vi "UDPrecieverShortLoop.vi"() -> ()   [LabVIEW 2012]
panel:
  out "Array":bool[][](array[boolean])
  out "size(s)":i32
  out "number":u32
  out "data pre process":u32
  out "packet in \nconstruction":u32
  out "data process":u32
  out "packet constructed":u32
  out "packet\nprocess":u32
  out "UDP reciever\nloop":u32
  out "start time":u32
  out "channel 11":u32[](graph)
  out "in 11":bool
  out "channel 10":u32[](graph)
  out "in 10":bool
  out "channel 9":u32[](graph)
  out "in 9":bool
  out "channel 8":u32[](graph)
  out "in 8":bool
  out "channel 7":u32[](graph)
  out "in 7":bool
  out "channel 6":u32[](graph)
  out "in 6":bool
  out "channel 5":u32[](graph)
  out "in 5":bool
  out "channel 4":u32[](graph)
  out "in 4":bool
  out "channel 3":u32[](graph)
  out "in 3":bool
  out "channel 2":u32[](graph)
  out "in 2":bool
  out "channel 1":u32[](graph)
  out "in 1":bool
  out "channel 0":u32[](graph)
  out "in 0":bool
  out "NumBins":u32
  out "Cnts/Bin":u32
  out "Prof/Hist":u32
  out "Sync":u32
  out "Channel":u32
  out "rTime":u32
  out "frameCntr":u32
  out "built packet array":string[](array[string])
  out "channel":u32
  out "Found Header":bool
  out "Raw Data Out":string
  out "error post-check":errorcluster
  out "End Reciever Error":errorcluster
  in  "stop reciever":bool
  out "port":u16
  out "error out post-read":errorcluster
  out "error out pre-read":errorcluster
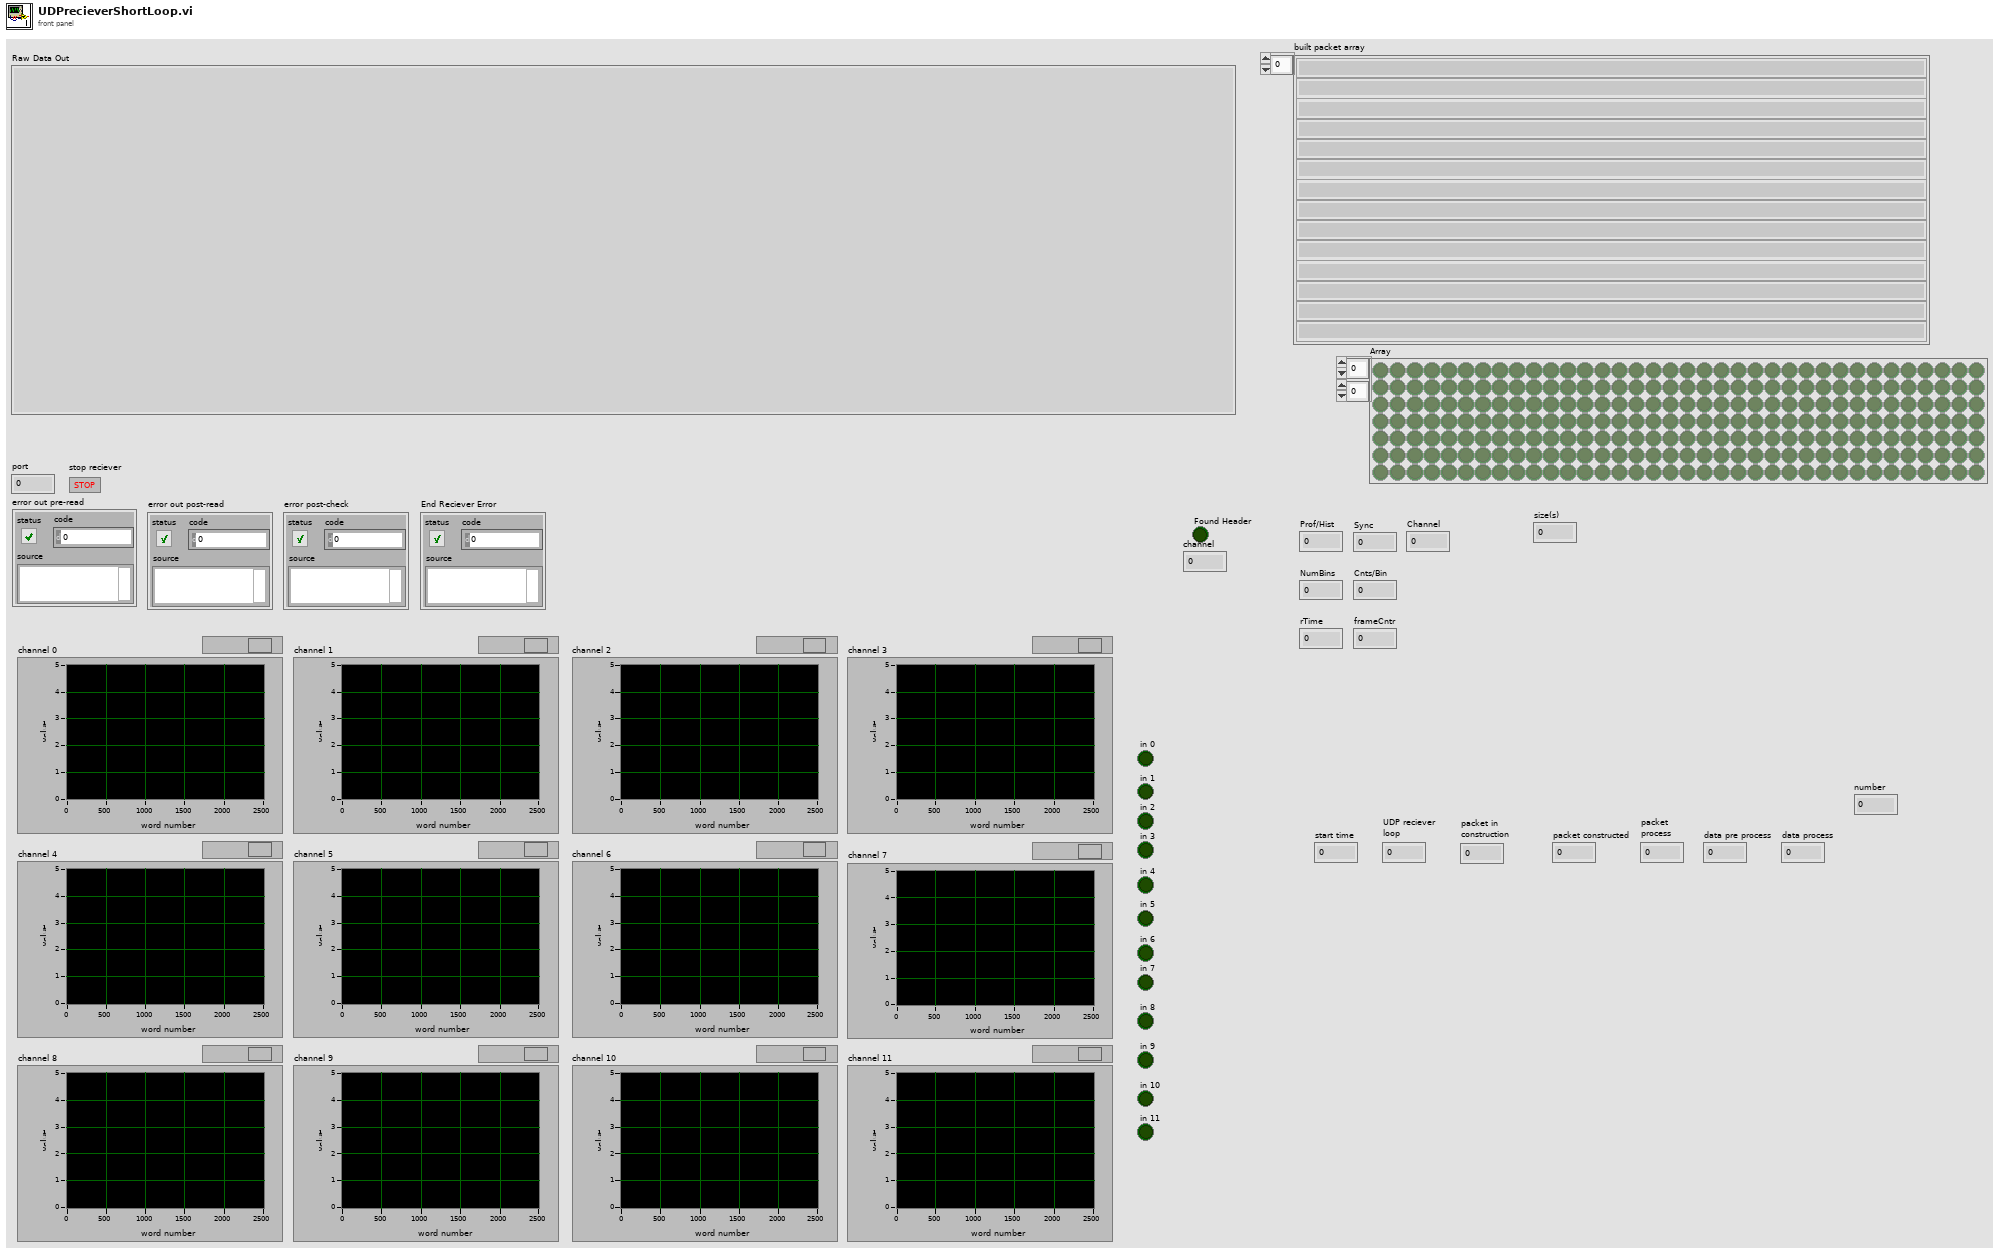
[diagram p1: front panel]
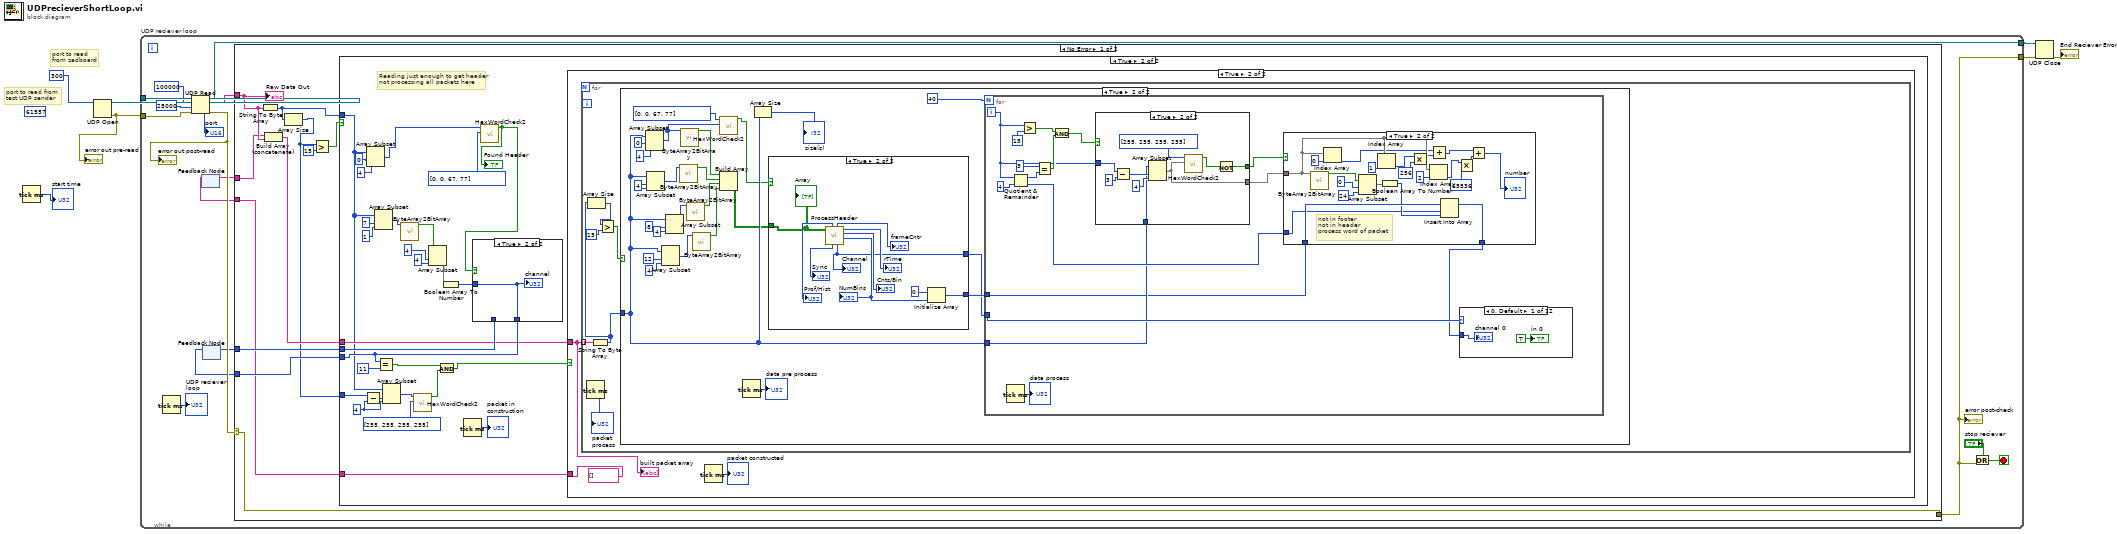
[diagram p0: block diagram]
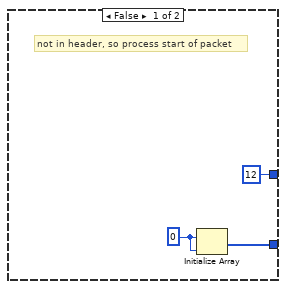
[diagram p5: hidden frame]
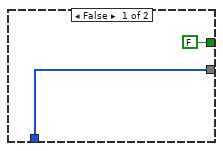
[diagram p6: hidden frame]
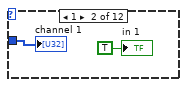
[diagram p7: hidden frame]
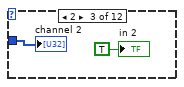
[diagram p8: hidden frame]
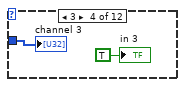
[diagram p9: hidden frame]
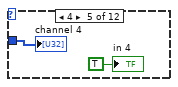
[diagram p10: hidden frame]
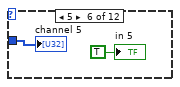
[diagram p11: hidden frame]
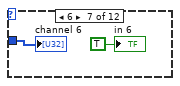
[diagram p12: hidden frame]
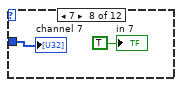
[diagram p13: hidden frame]
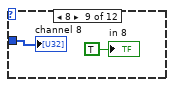
[diagram p14: hidden frame]
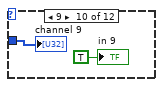
[diagram p15: hidden frame]
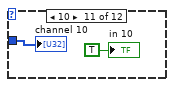
[diagram p16: hidden frame]
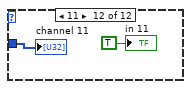
[diagram p17: hidden frame]
diagram:
  (unwired) u16 61557 ("port")
  # "port to read \nfrom zedboard"
  # "port to read from \ntest UDP sender"
  n1 = Tick Count (ms)() -> (millisecond timer value=→"start time":u32)
  n2 = UDP Open(11:u16 300 ("port")) -> (port=w6:refnum<k16>, 0:w3:errorcluster)  [unwired: 4 in, 1 out]
  "error out pre-read" <- w3
  n3 = while "UDP reciever loop" {
    tunnel: [w23] -> w7
    tunnel: w6 -> [w22]
    tunnel: [w14] -> w5
    tunnel: w3 -> [w19]
    stop <- w21 stop-if-true
    n4 = Tick Count (ms)() -> (millisecond timer value=→"UDP reciever\nloop":u32)
    n5 = UDP Read(connection ID=w22, max size (548)=100000, timeout ms (25000)=25000, 8:w19) -> (data out=w16:string, error out=w18:errorcluster, 3:w23:refnum<k16>, 4:→"port":u16)  [unwired: 1 out]
    "error out post-read" <- w18
    n6 = feedback #1() -> (w11:string[])  [unwired: 1 in]
    n7 = feedback #2() -> (w9:u32)  [unwired: 1 in]
    n8 = case shown="No Error" w18 {
      selector: w18 -> [w34 w189]
      tunnel: w16 -> [w33 _]
      tunnel: [w34 w189] -> w14
      tunnel: [w25 w188] -> w12
      tunnel: w11 -> [w32 w188]
      tunnel: [w29 w187] -> w10
      tunnel: w9 -> [w28 w187]
      frame No Error {
        n9 = String To Byte Array(string=w33) -> (unsigned byte array=w26:u8[])
        n10 = Build Array (concatenate)(w32, w33) -> (w27:string[])
        n11 = Array Size(array=w26) -> (size(s)=w24:i32)
        n12 = Greater?(x=w24, y=15) -> (0:w31:bool)
        n13 = case shown="True" w31 {
          tunnel: w26 -> [_ w46]
          tunnel: [w36 w50] -> w29
          tunnel: w28 -> [w36 w51]
          tunnel: w24 -> [_ w54]
          tunnel: w27 -> [w35 w48]
          tunnel: [w35 w47] -> w25
          frame False {
          }
          frame True {
            w56 = 4 ("length")
            # "Reading just enough to get header\nnot processing all packets here"
            n14 = Subtract(x=w54, y=w56) -> (x-y=w55:i32)
            n15 = Array Subset(array=w46, index=0, length=4) -> (w60:u8[])
            n16 = Array Subset(array=w46, index=7, length=1) -> (w43:u8[])
            n17 = Array Subset(array=w46, index=w55, length=w56) -> (w49:u8[])
            n18 = call "ByteArray2BitArray.vi"("array"=w43) -> ("Array"=w40:bool[])  [unwired: 10 in]
            n19 = call "HexWordCheck2.vi"("array"=u8[] [255, 255, 255, 255], "Input Array"=w49) -> ("Boolean"=w57:bool)  [unwired: 9 in]
            n20 = Array Subset(array=w40, index=4, length=4) -> (w38:bool[])
            n21 = Boolean Array To Number(Boolean array=w38) -> (number=w39:u32)
            n22 = Tick Count (ms)() -> (millisecond timer value=→"packet in \nconstruction":u32)
            n23 = call "HexWordCheck2.vi"("array"=u8[] [0, 0, 67, 77], "Input Array"=w60) -> ("Boolean"=w61:bool)  [unwired: 9 in]
            "Found Header" <- w61
            n24 = case shown="True" w61 {
              tunnel: [w185 w186] -> w50
              tunnel: w51 -> [w185 _]
              tunnel: w39 -> [_ w186]
              frame False {
              }
              frame True {
                "channel" <- w186
              }
            }
            n25 = Equal?(x=w50, y=u32 11) -> (x = y?=w53:bool)
            n26 = And(x=w53, y=w57) -> (x .and. y?=w58:bool)
            n27 = case shown="True" w58 {
              tunnel: w48 -> [w65 w67]
              tunnel: [w65 string[] []] -> w47
              frame False {
              }
              frame True {
                n28 = for {
                  tunnel: w67 -> [w74] mode=indexing
                  n29 = Tick Count (ms)() -> (millisecond timer value=→"packet\nprocess":u32)
                  n30 = String To Byte Array(string=w74) -> (unsigned byte array=w73:u8[])
                  n31 = Array Size(array=w73) -> (size(s)=w72:i32)
                  n32 = Greater?(x=w72, y=15) -> (0:w70:bool)
                  n33 = case shown="True" w70 {
                    tunnel: w73 -> [_ w82]
                    frame False {
                    }
                    frame True {
                      w87 = 4 ("length")
                      n34 = Array Subset(array=w82, index=0, length=4) -> (w97:u8[])
                      n35 = Array Subset(array=w82, index=w87, length=w87) -> (w83:u8[])
                      n36 = Array Subset(array=w82, index=12, length=4) -> (w96:u8[])
                      n37 = Array Subset(array=w82, index=8, length=4) -> (w84:u8[])
                      n38 = call "ByteArray2BitArray.vi"("array"=w83) -> ("Array"=w93:bool[])  [unwired: 10 in]
                      n39 = call "ByteArray2BitArray.vi"("array"=w97) -> ("Array"=w92:bool[])  [unwired: 10 in]
                      n40 = call "ByteArray2BitArray.vi"("array"=w84) -> ("Array"=w95:bool[])  [unwired: 10 in]
                      n41 = call "ByteArray2BitArray.vi"("array"=w96) -> ("Array"=w94:bool[])  [unwired: 10 in]
                      n42 = call "HexWordCheck2.vi"("array"=w97, "Input Array"=u8[] [0, 0, 67, 77] ("array")) -> ("Boolean"=w81:bool)  [unwired: 9 in]
                      n43 = Build Array(w92, w93, w95, w94) -> (w80:bool[][])
                      n44 = Tick Count (ms)() -> (millisecond timer value=→"data pre process":u32)
                      n45 = Array Size(array=w82) -> (size(s)=→"size(s)":i32)
                      n46 = case shown="True" w81 {
                        tunnel: w80 -> [_ w105]
                        tunnel: [w101 w104] -> w79
                        tunnel: [u32 12 ("Numeric 4") w102] -> w78
                        frame False {
                          w99 = u32 0 ("element")
                          # "not in header, so process start of packet"
                          n47 = Initialize Array(w99, w99) -> (w101:u32[])
                        }
                        frame True {
                          n48 = call "ProcessHeader.vi"("Array"=w105) -> ("Numeric"=w106:u32, "Numeric 7"=→"Cnts/Bin":u32, "Numeric 3"=→"rTime":u32, "Numeric 4"=w102:u32, "Numeric 2"=→"frameCntr":u32, "Numeric 5"=→"Sync":u32, "Numeric 6"=→"Prof/Hist":u32)  [unwired: 4 in]
                          "NumBins" <- w106
                          "Channel" <- w102
                          n49 = Initialize Array(u32 0 ("element"), w106) -> (w104:u32[])
                          "Array" <- w105
                        }
                      }
                      n50 = for {
                        N: 40 -> [_]
                        tunnel: w82 -> [w115]
                        tunnel: w79 -> [w114]
                        tunnel: w78 -> [w125]
                        i -> [w112]
                        n51 = Tick Count (ms)() -> (millisecond timer value=→"data process":u32)
                        n52 = Quotient & Remainder(x=w112, y=4) -> (x-y*floor(x/y)=w121:i32, floor(x/y)=w123:i32)
                        n53 = Greater?(x=w112, y=15 ("x")) -> (0:w120:bool)
                        n54 = Equal?(x=3, y=w121) -> (x = y?=w119:bool)
                        n55 = And(x=w120, y=w119) -> (x .and. y?=w118:bool)
                        n56 = case shown="True" w118 {
                          tunnel: w115 -> [w128 w134]
                          tunnel: [FALSE ("Boolean") w131] -> w116
                          tunnel: [w128 w133] -> w117
                          tunnel: w112 -> [_ w132]
                          frame False {
                          }
                          frame True {
                            n57 = Subtract(x=w132, y=3) -> (x-y=w137:i32)
                            n58 = Array Subset(array=w134, index=w137, length=4) -> (w133:u8[])
                            n59 = call "HexWordCheck2.vi"("array"=w133, "Input Array"=u8[] [255, 255, 255, 255] ("array")) -> ("Boolean"=w130:bool)  [unwired: 9 in]
                            n60 = Not(x=w130) -> (.not. x?=w131:bool)
                          }
                        }
                        n61 = case shown="True" w116 {
                          tunnel: w114 -> [w163 w184]
                          tunnel: w117 -> [_ w173]
                          tunnel: [w163 w178] -> w124
                          tunnel: w123 -> [_ w177]
                          frame False {
                          }
                          frame True {
                            # "not in footer \nnot in header\nprocess word of packet"
                            n62 = call "ByteArray2BitArray.vi"("array"=w173) -> ("Array"=w179:bool[])  [unwired: 10 in]
                            n63 = Index Array(array=w173, index=0) -> (element=w172:u8)
                            n64 = Array Subset(array=w179, index=0, length=24) -> (w181:bool[])
                            n65 = Index Array(array=w173, index=1) -> (element=w170:u8)
                            n66 = Boolean Array To Number(Boolean array=w181) -> (number=w180:u32)
                            n67 = Multiply(x=w170, y=256) -> (x*y=w171:i32)
                            n68 = Index Array(array=w173, index=2) -> (element=w166:u8)
                            n69 = Add(x=w172, y=w171) -> (x+y=w168:i32)
                            n70 = Insert Into Array(array=w184, index=w177, new element=w180) -> (w178:u32[])
                            n71 = Multiply(x=w166, y=65536) -> (x*y=w167:i32)
                            n72 = Add(x=w168, y=w167) -> (x+y=→"number":i32)
                          }
                        }
                        n73 = case shown="0, Default" w125 {
                          tunnel: w124 -> [w140 w142 w144 w146 w148 w150 w152 w154 w156 w158 w160 w162]
                          frame 0, Default {
                            "channel 0" <- w140
                            "in 0" <- TRUE ("in 11")
                          }
                          frame 1 {
                            "channel 1" <- w142
                            "in 1" <- TRUE ("in 11")
                          }
                          frame 2 {
                            "channel 2" <- w144
                            "in 2" <- TRUE ("in 11")
                          }
                          frame 3 {
                            "channel 3" <- w146
                            "in 3" <- TRUE ("in 11")
                          }
                          frame 4 {
                            "channel 4" <- w148
                            "in 4" <- TRUE ("in 11")
                          }
                          frame 5 {
                            "channel 5" <- w150
                            "in 5" <- TRUE ("in 11")
                          }
                          frame 6 {
                            "channel 6" <- w152
                            "in 6" <- TRUE ("in 11")
                          }
                          frame 7 {
                            "channel 7" <- w154
                            "in 7" <- TRUE ("in 11")
                          }
                          frame 8 {
                            "channel 8" <- w156
                            "in 8" <- TRUE ("in 11")
                          }
                          frame 9 {
                            "channel 9" <- w158
                            "in 9" <- TRUE ("in 11")
                          }
                          frame 10 {
                            "channel 10" <- w160
                            "in 10" <- TRUE ("in 11")
                          }
                          frame 11 {
                            "channel 11" <- w162
                            "in 11" <- TRUE ("in 11")
                          }
                        }
                      }
                    }
                  }
                }
                n74 = Tick Count (ms)() -> (millisecond timer value=→"packet constructed":u32)
                "built packet array" <- w67
              }
            }
          }
        }
        "Raw Data Out" <- w33
      }
      frame Error {
      }
    }
    "error post-check" <- w14
    n75 = feedback-in #1(w12) -> ()
    n76 = feedback-in #2(w10) -> ()
    n77 = Or(x="stop reciever", y=w14) -> (x .or. y?=w21:bool)
  }
  n78 = UDP Close(connection ID=w7, 8:w5) -> (error out=→"End Reciever Error":errorcluster)  [unwired: 1 out]
